vi "rc_initialize barometer.vi"(8 "error in (no error)":errorcluster, 10 "filter":u32(ring), 11 "oversample":u32(ring)) -> (0 "error out":errorcluster, 3 "function return":i32)   [LabVIEW 2014, in "libroboticscape.lvlib"]
doc: "int initialize_barometer(bmp_oversample_t oversample, bmp_filter_t filter);\n\nint initialize_barometer(int oversample, int filter);"
uses:
  libroboticscape.lvlib
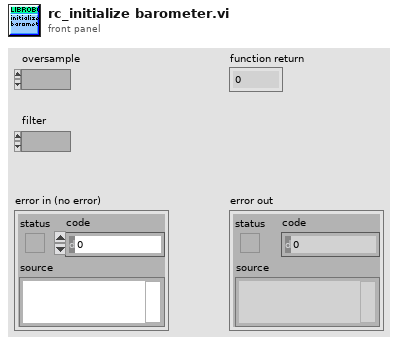
[diagram p1: front panel]
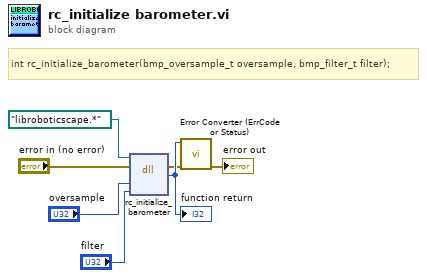
[diagram p0: block diagram]
diagram:
  # "int rc_initialize_barometer(bmp_oversample_t oversample, bmp_filter_t filter);"
  n1 = dll-call lib="C:/Users/ktalke/Documents/Robotics-Cape-Master-Jessie/Libroboticscape-Master-Jessie/libroboticscape.so" fn="rc_initialize_barometer"(path in=path "libroboticscape.*", error in="error in (no error)", "oversample"="oversample", "filter"="filter") -> (error out=w3:errorcluster, "return type"=w7:i32)  [unwired: 3 in, 1 out]
  "function return" <- w7
  n2 = call "Error Converter (ErrCode or Status).vi"("error in (no error)"=w3, "error code"=w7) -> ("error out"=→"error out":errorcluster)  [unwired: 9 in]
